vi "ADC Example LaunchPad.vi"() -> ()   [LabVIEW 2011]
panel:
  in  "stop":bool
  in  "Dial Time Interval (ms)":u32(knob)=1009 scale=0.0..2000.0
  in  "Ring":u16(ring)=8 items=["Analog Input 1(P1.4)"=4, "Analog Input 2(P1.5)"=5, "Analog Input 3(P1.7)"=7, "Temperature(deg C)"=8, "Voltage Source (Vcc)"=9]
  out "Meter":dbl(knob) scale=0.0..50.0
  out "CurrentPath":path=path "C:/Documents and Settings/TGI0362/My Documents/xUserData/LabVIEW_8.x/cmDVT_Factory-BBU-R5"
  out "new picture":picture
  # "ADC10 example \nwtih adjustable sampling time delay"
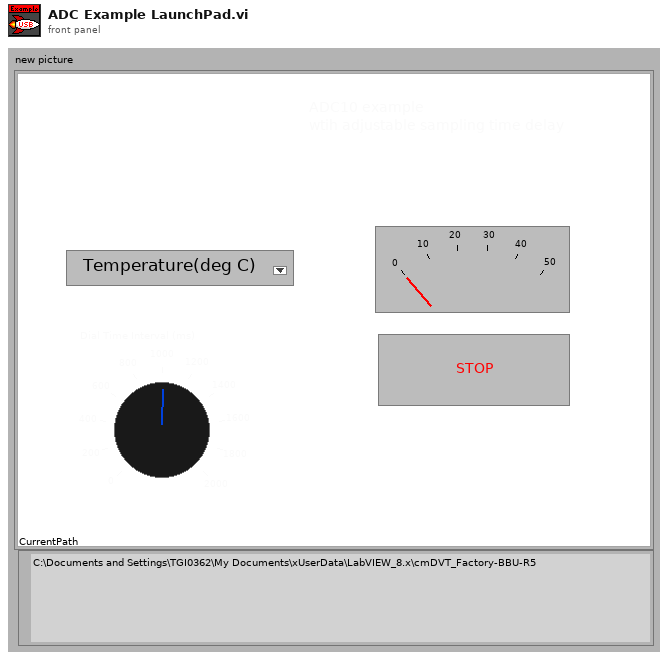
[diagram p1: front panel]
types:
  T1 = typedef "imagedata.ctl" = cluster{"image type":i32, "image depth":i32, "image":u8[], "mask":u8[], "colors":u32[], "Rectangle":cluster{"left":i16, "top":i16, "right":i16, "bottom":i16}}
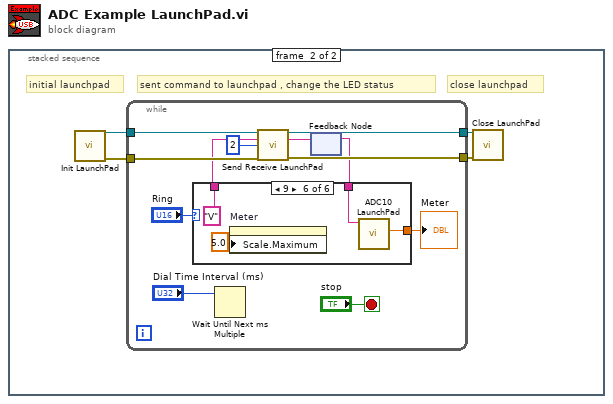
[diagram p0: block diagram]
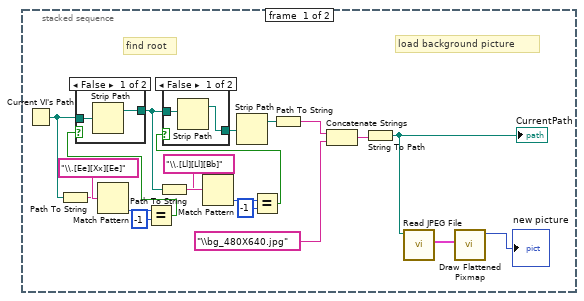
[diagram p2: hidden frame]
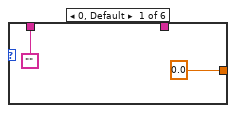
[diagram p5: hidden frame]
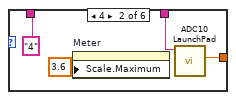
[diagram p6: hidden frame]
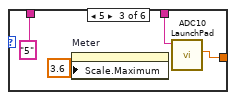
[diagram p7: hidden frame]
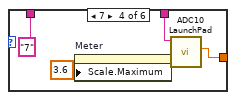
[diagram p8: hidden frame]
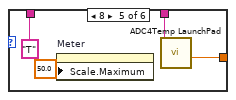
[diagram p9: hidden frame]
diagram:
  n1 = stacked-sequence {
    frame #0 {
      # "load background picture"
      # "find root"
      n2 = Current VI's Path() -> (path=w9:path)
      n3 = Path To String(path=w9) -> (string=w8:string)
      n4 = Match Pattern(string=w8, regular expression="\\.[Ee][Xx][Ee]") -> (offset past match=w6:i32)  [unwired: 1 in, 3 out]
      n5 = Equal?(x=w6, y=-1) -> (x = y?=w18:bool)
      n6 = case shown="False" w18 {
        tunnel: [w24 w26] -> w15
        tunnel: w9 -> [w25 w26]
        frame False {
          n7 = Strip Path(path=w25) -> (stripped path=w24:path)  [unwired: 1 out]
        }
        frame True {
        }
      }
      n8 = Path To String(path=w15) -> (string=w12:string)
      n9 = Match Pattern(string=w12, regular expression="\\.[Ll][Ll][Bb]") -> (offset past match=w14:i32)  [unwired: 1 in, 3 out]
      n10 = Equal?(x=w14, y=-1) -> (x = y?=w17:bool)
      n11 = case shown="False" w17 {
        tunnel: [w21 w23] -> w16
        tunnel: w15 -> [w22 w23]
        frame False {
          n12 = Strip Path(path=w22) -> (stripped path=w21:path)  [unwired: 1 out]
        }
        frame True {
        }
      }
      n13 = Strip Path(path=w16) -> (stripped path=w5:path)  [unwired: 1 out]
      n14 = Path To String(path=w5) -> (string=w2:string)
      n15 = Concatenate Strings(w2, "\\bg_480X640.jpg") -> (w3:string)
      n16 = String To Path(string=w3) -> (path=w1:path)
      "CurrentPath" <- w1
      n17 = call <vilib>:"Read JPEG File.vi"("path to JPEG file"=w1) -> ("image data"=w19:T1)  [unwired: 8 in, 2 out]
      n18 = call <vilib>:"Draw Flattened Pixmap.vi"("image data"=w19) -> ("new picture"=→"new picture":picture)  [unwired: 8 in]
    }
    frame #1 {
      # "close launchpad"
      # "sent command to launchpad , change the LED status"
      # "initial launchpad"
      n19 = call "Init LaunchPad.vi"() -> ("error out"=w27:errorcluster, "VISA resource name out"=w30:refnum<visa-resource-name>)  [unwired: 10 in]
      n20 = while {
        tunnel: w30 -> [w42]
        tunnel: [w41] -> w29
        tunnel: [w40] -> w28
        tunnel: w27 -> [w39]
        stop <- "stop" stop-if-true
        n21 = Wait Until Next ms Multiple(millisecond multiple="Dial Time Interval (ms)") -> ()  [unwired: 1 out]
        n22 = feedback #1() -> (w32:string)  [unwired: 1 in]
        n23 = case shown="9" "Ring" {
          tunnel: ["" "4" "5" "7" "T" "V"] -> w35
          tunnel: w32 -> [_ w46 w50 w54 w59 w63]
          tunnel: [0.0 ("Temp (deg C)") w47 w51 w55 w58 w62] -> w31
          frame 0, Default {
          }
          frame 4 {
            n24 = property on="Meter" class="Knob (strict)"("Scale.Maximum"=3.6 ("Scale.Range:Maximum")) -> ()  [unwired: 2 in, 2 out]
            n25 = call "ADC10 LaunchPad.vi"("string"=w46) -> ("ADC10 (Volt)"=w47:dbl)  [unwired: 9 in, 1 out]
          }
          frame 5 {
            n26 = property on="Meter" class="Knob (strict)"("Scale.Maximum"=3.6 ("Scale.Range:Maximum")) -> ()  [unwired: 2 in, 2 out]
            n27 = call "ADC10 LaunchPad.vi"("string"=w50) -> ("ADC10 (Volt)"=w51:dbl)  [unwired: 9 in, 1 out]
          }
          frame 7 {
            n28 = property on="Meter" class="Knob (strict)"("Scale.Maximum"=3.6 ("Scale.Range:Maximum")) -> ()  [unwired: 2 in, 2 out]
            n29 = call "ADC10 LaunchPad.vi"("string"=w54) -> ("ADC10 (Volt)"=w55:dbl)  [unwired: 9 in, 1 out]
          }
          frame 8 {
            n30 = property on="Meter" class="Knob (strict)"("Scale.Maximum"=50.0 ("Scale.Range:Maximum")) -> ()  [unwired: 2 in, 2 out]
            n31 = call "ADC4Temp LaunchPad.vi"("string"=w59) -> ("Temp (deg C)"=w58:dbl)  [unwired: 8 in, 2 out]
          }
          frame 9 {
            n32 = property on="Meter" class="Knob (strict)"("Scale.Maximum"=5.0 ("Scale.Range:Maximum")) -> ()  [unwired: 2 in, 2 out]
            n33 = call "ADC10 LaunchPad.vi"("string"=w63) -> ("ADC10 (Volt)"=w62:dbl)  [unwired: 9 in, 1 out]
          }
        }
        "Meter" <- w31
        n34 = call "Send Receive LaunchPad.vi"("VISA resource"=w42, "write buffer"=w35, "Bytes To Read (0)"=u8 2, "error in"=w39) -> ("VISA resource 2"=w41:refnum<visa-resource-name>, "Read Buffer"=w33:string, "error out"=w40:errorcluster)  [unwired: 9 in]
        n35 = feedback-in #1(w33) -> ()
      }
      n36 = call "Close LaunchPad.vi"("VISA resource name"=w29, "error in"=w28) -> ()  [unwired: 13 in, 1 out]
    }
  }
